vi "Module Top Level.vi"(8 "error in":errorcluster) -> (0 "error out":errorcluster)   [LabVIEW 2018, in "UDP Reader.lvlib"]
doc: "This is the top level VI for this module. It uses a queue for communications and is stopped user a user event. The general architecture is similar to a simple queued message handler.\n\nThe VIs associated with this module are organized in a LabVIEW Library."
uses:
  UDP Reader.lvlib
  Private Controls/Host Comms Data.ctl
  Private Controls/Module Data.ctl
  Private Controls/Module Action.ctl
  Top Level/Shared Controls/cRIOData.ctl
  Modules/Testing UI 1/Private Controls/APU & ECU Controls.ctl
  Modules/Testing UI 1/Public Controls/Bleed-Fuel-ECS Controls.ctl
  Modules/Testing UI 3/Private Controls/Cutoff Frequency.ctl
  cac91517-d732-413a-8e65-b4ff920fc073.vi
  Modules/Testing UI 1/Testing UI 1.lvlib
  Modules/Testing UI 3/Testing UI 3.lvlib
  RT - Instrument IO/Outputs.lvlib
  RT - Vibration/Vibration.lvlib
panel:
  out "Numeric Control":i32
  out "Connected?":bool
  # "UDP Reader"
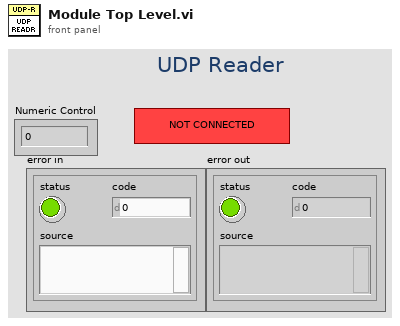
[diagram p1: front panel]
types:
  T1 = typedef "UDP Reader.lvlib/Host Comms Data.ctl" = cluster{"Connected?":bool, "connection ID":refnum<k16>}
  T2 = typedef "cRIOData.ctl" = cluster{"APU & ECU Controls":T3, "APU Start":bool, "Bleed Fuel ECS Controls":T4, "FuelPressureReg":dbl, "ECS Demand":dbl, "Accel Sensitivities":dbl[], "Accel Filters":T5[], "ShuntRelay":bool, "Waterfall Select":u8}
  T3 = typedef "Testing UI 1.lvlib/APU & ECU Controls.ctl" = cluster{"02.01.9485.06":bool, "FuelPump":bool, "02.00.9485.01":bool, "02.00.9485.02":bool, "02.00.9485.03":bool, "02.00.9485.05":bool, "02.00.9485.04":bool, "02.00.9485.00":bool, "02.00.9485.07":bool, "02.01.9485.00":bool, "02.01.9485.01":bool}
  T4 = typedef "Testing UI 1.lvlib/Bleed-Fuel-ECS Controls.ctl" = cluster{"Coarse_RC":bool, "Coarse_RO":bool, "Bleed-Fine-Knob":dbl, "Bleed-Coarse-Knob":dbl}
  T5 = typedef "Testing UI 3.lvlib/Cutoff Frequency.ctl" = cluster{"LP Passband":dbl, "HP Stopband":dbl, "LP Stopband":dbl, "HP Passband":dbl}
  T6 = typedef "UDP Reader.lvlib/Module Data.ctl" = cluster{"Data":variant, "Action":T7}
  T7 = typedef "UDP Reader.lvlib/Module Action.ctl" = enum16{"Init", "Read", "Error"}
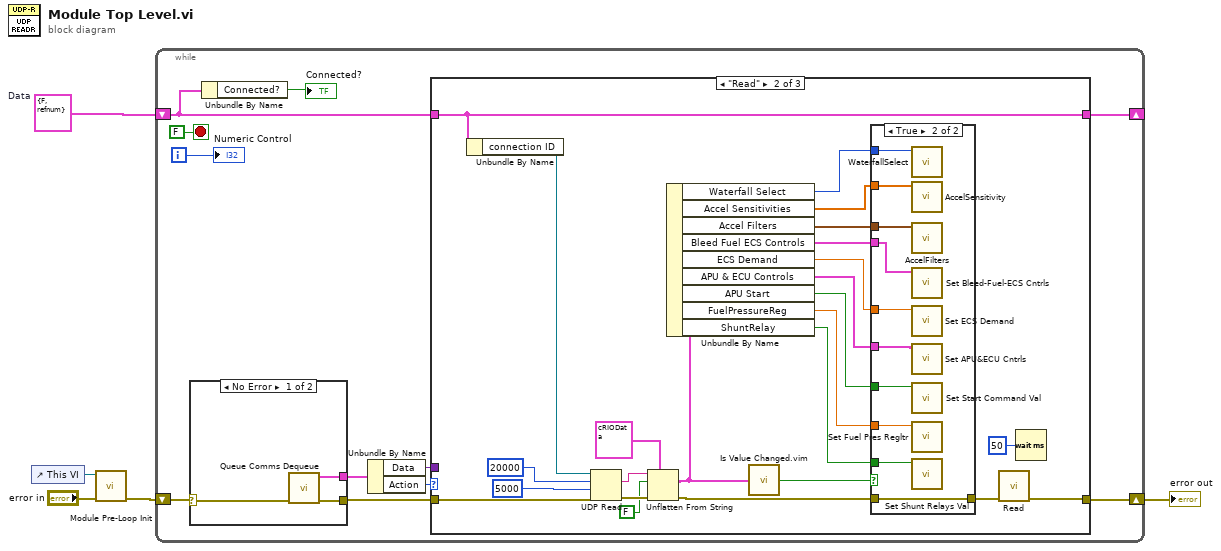
[diagram p0: block diagram]
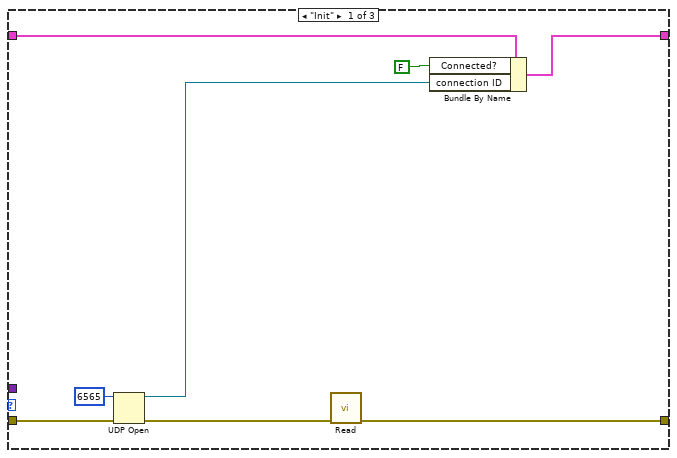
[diagram p2: hidden frame]
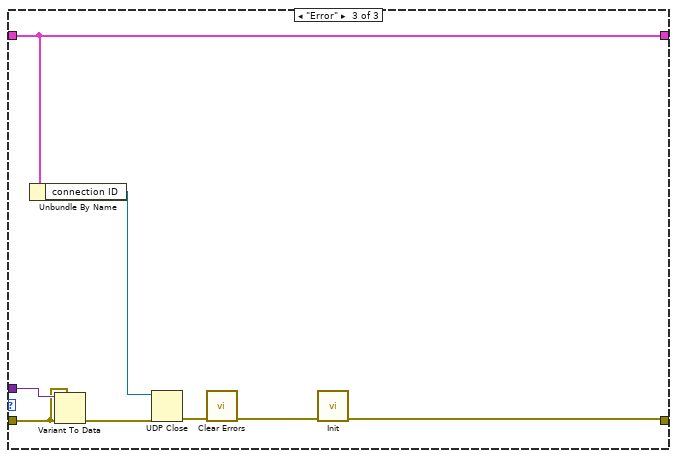
[diagram p4: hidden frame]
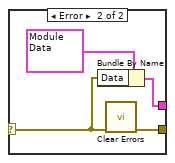
[diagram p5: hidden frame]
diagram:
  w2 = T1 {"Connected?"=FALSE, "connection ID"=refnum}  # Data
  n1 = control-ref of="This VI"() -> (w5:refnum<vi>)
  n2 = call "Module Pre-Loop Init.vi"("error in (no error)"="error in", "Top Level VI Ref in"=w5) -> ("error out"=w1:errorcluster)  [unwired: 9 in]
  n3 = while {
    shift-right: [w12] -> w3
    shift-left: w1 -> [w11]
    shift-right: [w10] -> _
    shift-left: w2 -> [w9]
    i -> [w6]
    stop <- FALSE stop-if-true
    n4 = case shown="No Error" w11 {
      selector: w11 -> [w69 w72]
      tunnel: [w70 w73] -> w16
      tunnel: [w68 w71] -> w13
      frame No Error {
        n5 = call "Queue Comms Dequeue.vi"("error in (no error)"=w69) -> ("error out"=w68:errorcluster, "element"=w70:T6)  [unwired: 9 in]
      }
      frame Error {
        n6 = Bundle By Name(cluster=T6 {"Data"=variant, "Action"=enum."Error"} ("element"), "Data"=w72) -> (w73:T6)
        n7 = call <vilib>:"Clear Errors.vi"("error in (no error)"=w72) -> ("error out"=w71:errorcluster)  [unwired: 5 in, 1 out]
      }
    }
    n8 = Unbundle By Name(w9) -> ("Connected?"=→"Connected?":bool)
    n9 = Unbundle By Name(w16) -> ("Data"=w14:variant, "Action"=w15:T7)
    n10 = case shown="\"Read\"" w15 {
      tunnel: w14 -> [_ _ w67]
      tunnel: w13 -> [w21 w46 w66]
      tunnel: [w17 w43 w65] -> w12
      tunnel: [w24 w48 w63] -> w10
      tunnel: w9 -> [w23 w48 w63]
      frame "Init" {
        n11 = UDP Open(8:w21, 11:u16 6565 ("port")) -> (port=w19:refnum<k16>, 0:w18:errorcluster)  [unwired: 3 in, 1 out]
        n12 = call "Read.vi"("error in"=w18) -> ("error out"=w17:errorcluster)  [unwired: 10 in]
        n13 = Bundle By Name(cluster=w23, "Connected?"=FALSE, "connection ID"=w19) -> (w24:T1)
      }
      frame "Read" {
        n14 = Unbundle By Name(w48) -> ("connection ID"=w47:refnum<k16>)
        n15 = UDP Read(connection ID=w47, max size (548)=20000, timeout ms (25000)=5000, 8:w46) -> (data out=w29:string, error out=w30:errorcluster)  [unwired: 3 out]
        n16 = Unflatten From String(type=T2 {"APU & ECU Controls"={"02.01.9485.06"=FALSE, "FuelPump"=FALSE, "02.00.9485.01"=FALSE, "02.00.9485.02"=FALSE, "02.00.9485.03"=FALSE, "02.00.9485.05"=FALSE, "02.00.9485.04"=FALSE, "02.00.9485.00"=FALSE, "02.00.9485.07"=FALSE, "02.01.9485.00"=FALSE, "02.01.9485.01"=FALSE}, "APU Start"=FALSE, "Bleed Fuel ECS Controls"={"Coarse_RC"=FALSE, "Coarse_RO"=FALSE, "Bleed-Fine-Knob"=0.0, "Bleed-Coarse-Knob"=0.0}, "FuelPressureReg"=0.0, "ECS Demand"=0.0, "Accel Sensitivities"=[], "Accel Filters"=[], "ShuntRelay"=FALSE, "Waterfall Select"=0} ("cRIO Data"), binary string=w29, data includes array or string size? (T)=FALSE, error in (no error)=w30) -> (value=w26:T2, error out=w25:errorcluster)  [unwired: 1 in, 1 out]
        n17 = Unbundle By Name(w26) -> ("Waterfall Select"=w31:u8, "Accel Sensitivities"=w34:dbl[], "Accel Filters"=w42:T5[], "Bleed Fuel ECS Controls"=w41:T4, "ECS Demand"=w39:dbl, "APU & ECU Controls"=w38:T3, "APU Start"=w37:bool, "FuelPressureReg"=w36:dbl, "ShuntRelay"=w35:bool)
        n18 = call "Is Value Changed.vim"("value"=w26) -> ("changed or first call?"=w45:bool)
        n19 = case shown="True" w45 {
          tunnel: w25 -> [w49 w59]
          tunnel: [w49 w59] -> w44
          tunnel: w42 -> [_ w51]
          tunnel: w41 -> [_ w58]
          tunnel: w39 -> [_ w57]
          tunnel: w38 -> [_ w56]
          tunnel: w37 -> [_ w55]
          tunnel: w36 -> [_ w54]
          tunnel: w35 -> [_ w53]
          tunnel: w34 -> [_ w52]
          tunnel: w31 -> [_ w50]
          frame False {
          }
          frame True {
            n20 = call "WaterfallSelect.vi"("WaterfallSelect(0-4)"=w50) -> ()  [unwired: 10 in, 1 out]
            n21 = call "AccelSensitivity.vi"("Accel Sensistivity"=w52) -> ()  [unwired: 10 in, 1 out]
            n22 = call "AccelFilters.vi"("Cutoff Frequncies"=w51) -> ()  [unwired: 10 in, 1 out]
            n23 = call "Set Bleed-Fuel-ECS Cntrls.vi"("Bleed-Fuel-ECS Controls"=w58) -> ()  [unwired: 10 in, 1 out]
            n24 = call "Set ECS Demand.vi"("ECS Demand"=w57) -> ()  [unwired: 10 in, 1 out]
            n25 = call "Set APU&ECU Cntrls.vi"("APU & ECU Controls"=w56) -> ()  [unwired: 10 in, 1 out]
            n26 = call "Set Start Command Val.vi"("Value"=w55) -> ()  [unwired: 10 in, 1 out]
            n27 = call "Set Fuel Pres Regltr.vi"("FuelPressureReg"=w54) -> ()  [unwired: 10 in, 1 out]
            n28 = call "Set Shunt Relays Val.vi"("Value"=w53) -> ()  [unwired: 10 in, 1 out]
          }
        }
        n29 = call "Read.vi"("error in"=w44) -> ("error out"=w43:errorcluster)  [unwired: 10 in]
        n30 = Wait (ms)(milliseconds to wait=u32 50) -> ()  [unwired: 1 out]
      }
      frame "Error" {
        n31 = Unbundle By Name(w63) -> ("connection ID"=w62:refnum<k16>)
        n32 = Variant To Data(error in=w66, type=w66, Variant=w67) -> (error out=w64:errorcluster)  [unwired: 1 out]
        n33 = UDP Close(connection ID=w62, 8:w64) -> (error out=w61:errorcluster)  [unwired: 1 out]
        n34 = call <vilib>:"Clear Errors.vi"("error in (no error)"=w61) -> ("error out"=w60:errorcluster)  [unwired: 5 in, 1 out]
        n35 = call "Init.vi"("error in"=w60) -> ("error out"=w65:errorcluster)  [unwired: 10 in]
      }
    }
    "Numeric Control" <- w6
  }
  "error out" <- w3
